vi "Compile Routing Channels.vi"(8 "error in (no error)":errorcluster, 10 "Alias Mapping":T1, 11 "Device Ref in":T5 format="%.0x") -> (0 "error out":errorcluster, 2 "Routing Channels Configuration":T2[](array[typedef]), 3 "Device Ref out":T5 format="%.0x")   [LabVIEW 2017, in "Routing and Faulting System Explorer.lvlib"]
uses:
  Routing and Faulting System Explorer.lvlib
  <vilib>/NI Veristand/Custom Device API/Custom Device Item Ref.ctl
  Shared/Routing Channel Configuration.ctl
  Shared/Value-Connections Map.ctl
  Shared/Connection.ctl
  Shared/Alias Mapping.ctl
  Shared/Constants.vi
  <vilib>/NI Veristand/Custom Device Tools/Custom Device Utility Library/NI VeriStand - Search for Item by Name.vi
  <vilib>/NI Veristand/Custom Device Tools/Custom Device Utility Library/Custom Device Utility Library.lvlib
  Shared/Routing and Faulting Shared.lvlib
  Scripting/Switch Scripting.lvlib
  <vilib>/NI VeriStand/Custom Device API/Custom Device API.lvlib
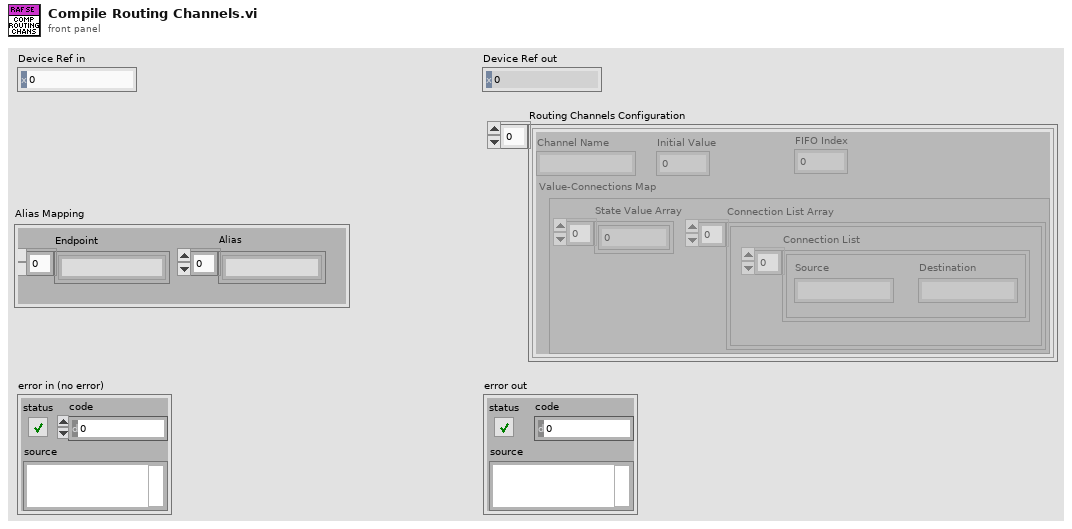
[diagram p1: front panel]
types:
  T1 = typedef "Routing and Faulting Shared.lvlib/Alias Mapping.ctl" = cluster{"Endpoint":string[], "Alias":string[]}
  T2 = typedef "Routing and Faulting Shared.lvlib/Routing Channel Configuration.ctl" = cluster{"Channel Name":string, "Initial Value":dbl, "FIFO Index":i32, "Value-Connections Map":T3}
  T3 = typedef "Routing and Faulting Shared.lvlib/Value-Connections Map.ctl" = cluster{"State Value Array":i32[], "Connection List Array":cluster{"Connection List":T4[]}[]}
  T4 = typedef "Routing and Faulting Shared.lvlib/Connection.ctl" = cluster{"Source":string, "Destination":string}
  T5 = typedef "Custom Device API.lvlib/Custom Device Item Ref.ctl" = u64
  T6 = typedef "Routing and Faulting Shared.lvlib/Channel States.ctl" = T7[]
  T7 = typedef "Routing and Faulting Shared.lvlib/Routing State.ctl" = cluster{"Name":string, "Description":string, "Value":i32, "Connection List":T4[]}
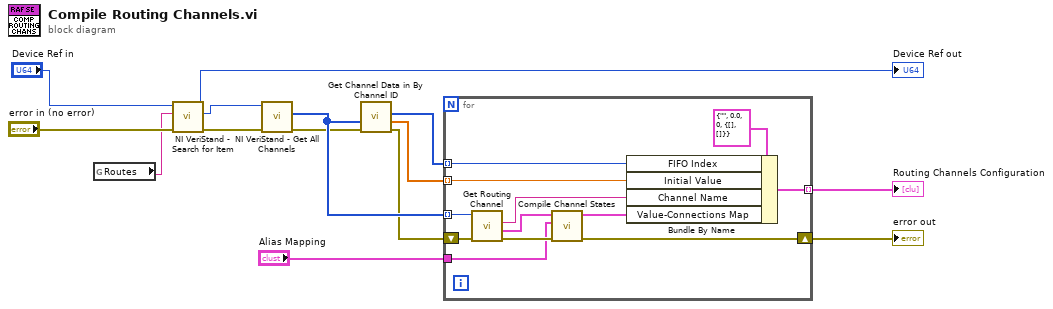
[diagram p0: block diagram]
diagram:
  n1 = global read "Constants.vi" "Routes"() -> (w2:string)
  n2 = call-poly <vilib>:"NI VeriStand - Search for Item.vi"("error in"="error in (no error)", "Item Name"=w2, "Section Ref in"="Device Ref in") -> ("error out"=w7:errorcluster, "Item Ref"=w6:T5, "Section Ref out"=→"Device Ref out":T5)  [unwired: 5 in, 1 out]
  n3 = call <vilib>:"NI VeriStand - Get All Channels.vi"("error in"=w7, "Section Ref in"=w6) -> ("error out"=w8:errorcluster, "Channel Refs"=w9:T5[])  [unwired: 6 in, 2 out]
  n4 = call "Get Channel Data in By Channel ID.vi"("error in (no error)"=w8, "Channel IDs"=w9) -> ("error out"=w5:errorcluster, "default values"=w3:dbl[], "FIFO indexes"=w4:i32[])  [unwired: 6 in, 1 out]
  n5 = for {
    tunnel: w9 -> [w26] mode=indexing
    tunnel: w3 -> [w21] mode=indexing
    tunnel: w4 -> [w24] mode=indexing
    shift-right: [w18] -> w13
    shift-left: w5 -> [w22]
    tunnel: [w20] -> w10 mode=indexing
    tunnel: "Alias Mapping" -> [w15]
    n6 = call "Get Routing Channel.vi"("error in (no error)"=w22, "Channel Ref in"=w26) -> ("error out"=w19:errorcluster, "Channel States"=w17:T6, "Channel Name"=w23:string)  [unwired: 5 in, 2 out]
    n7 = call "Compile Channel States.vi"("error in (no error)"=w19, "Alias Mapping"=w15, "Channel States"=w17) -> ("error out"=w18:errorcluster, "Value-Connections Map"=w16:T3)  [unwired: 7 in]
    n8 = Bundle By Name(cluster=T2 {"Channel Name"="", "Initial Value"=0.0, "FIFO Index"=0, "Value-Connections Map"={"State Value Array"=[], "Connection List Array"=[]}} ("Routing Channel Configuration"), "FIFO Index"=w24, "Initial Value"=w21, "Channel Name"=w23, "Value-Connections Map"=w16) -> (w20:T2)
  }
  "error out" <- w13
  "Routing Channels Configuration" <- w10
